vi "Komponenten setzen.vi"(8 "error in (no error)":errorcluster caption="Fehler (Eingang, kein Fehler)", 10 "Komponenten":T1[](array[typedef]) {"Konzentration SOLL" format="%#.4f"; "Konzentration IST" format="%#.4f"; "Genauigkeit" format="%#.1f"}) -> (0 "error out":errorcluster caption="Fehler (Ausgang)", 2 "Index":i32[](array[numeric]), 3 "found":bool[](array[boolean]))   [LabVIEW 2020, in "System Einstellungen V2.lvlib"]
uses:
  System Einstellungen V2.lvlib
  Gasflaschenkomponente.ctl
  FT-IR/FGV FT-IR Gasliste Aktionen.ctl
  FT-IR/FT-IR.lvlib
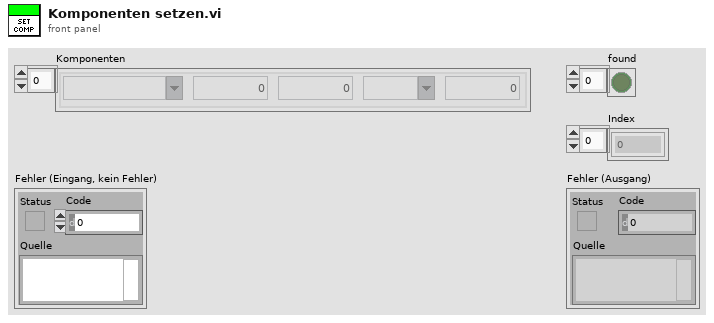
[diagram p1: front panel]
types:
  T1 = typedef "System Einstellungen V2.lvlib/Gasflaschenkomponente.ctl" = cluster{"Gasauswahl":string, "Konzentration SOLL":dbl, "Konzentration IST":dbl, "Einheit":string, "Genauigkeit":dbl}
  T2 = typedef "FT-IR.lvlib/FGV FT-IR Gasliste Aktionen.ctl" = enum16{"lesen", "Gasliste FT-IR", "Gasliste ausgelesen", "laden", "speichern", "löschen"}
  T3 = typedef "String - Ausgabefeld.ctl" = string
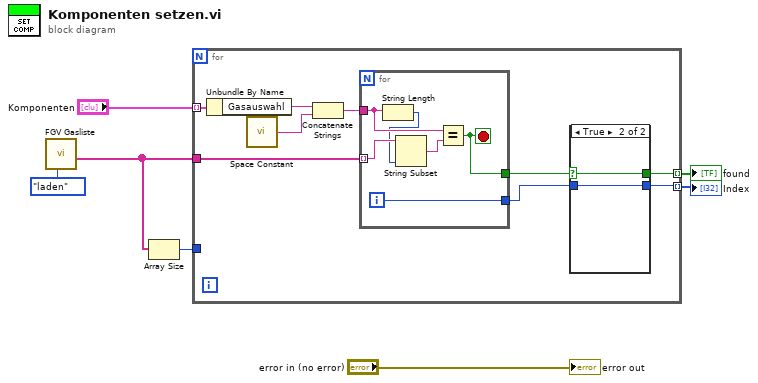
[diagram p0: block diagram]
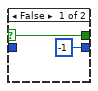
[diagram p2: hidden frame]
diagram:
  n1 = call "FGV Gasliste.vi"("Aktionen"=FGV_FT-IR_Gasliste_Aktionen."laden") -> ("Aktuelle Gasliste gesamt"=w4:T3[])  [unwired: 8 in, 2 out]
  n2 = Array Size(array=w4) -> (size(s)=w3:i32)
  n3 = for {
    tunnel: w4 -> [w16]
    tunnel: "Komponenten" -> [w15] mode=indexing
    tunnel: w3 -> [_]
    tunnel: [w12] -> w2 mode=indexing
    tunnel: [w11] -> w1 mode=indexing
    n4 = Unbundle By Name(w15) -> ("Gasauswahl"=w14:string)
    n5 = call <vilib>:"Space Constant.vi"() -> ("String"=w9:string)
    n6 = Concatenate Strings(w14, w9) -> (w10:string)
    n7 = for {
      tunnel: w16 -> [w23] mode=indexing
      tunnel: w10 -> [w24]
      tunnel: [w26] -> w8
      tunnel: [w25] -> w13
      i -> [w25]
      stop <- w26 stop-if-true
      n8 = String Length(string=w24) -> (length=w21:i32)
      n9 = String Subset(string=w23, length (rest)=w21) -> (substring=w22:T3)  [unwired: 1 in]
      n10 = Equal?(x=w24, y=w22) -> (x = y?=w26:bool)
    }
    n11 = case shown="True" w8 {
      selector: w8 -> [w17 w19]
      tunnel: w13 -> [_ w20]
      tunnel: [w17 w19] -> w12
      tunnel: [-1 w20] -> w11
      frame False {
      }
      frame True {
      }
    }
  }
  "found" <- w2
  "Index" <- w1
  "error out" <- "error in (no error)"
